vi "Write Results.vi"(8 "error in (no error)":errorcluster, 10 "Results":refnum<class "Acquired Result.lvclass">[](array[class]), 11 "Combined Result in":refnum<class "Combined Result.lvclass">) -> (0 "error out":errorcluster, 3 "Combined Result out":refnum<class "Combined Result.lvclass">)   [LabVIEW 2021, in "Combined Result.lvclass"]
uses:
  Combined Result.lvclass
  Acquired Result/Acquired Result.lvclass
  Combined Result.lvclass/Combined Result.ctl
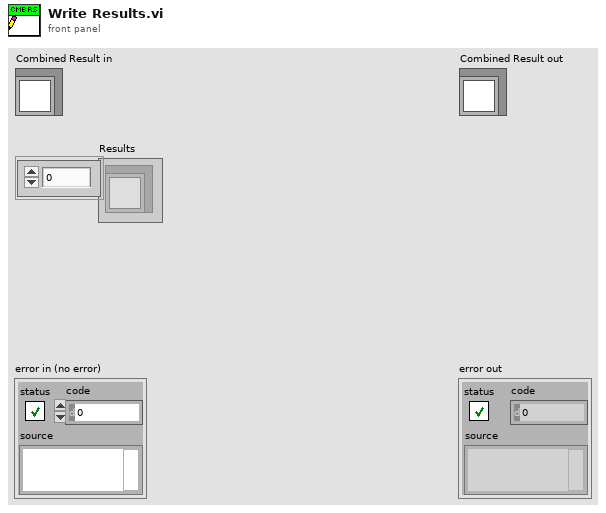
[diagram p1: front panel]
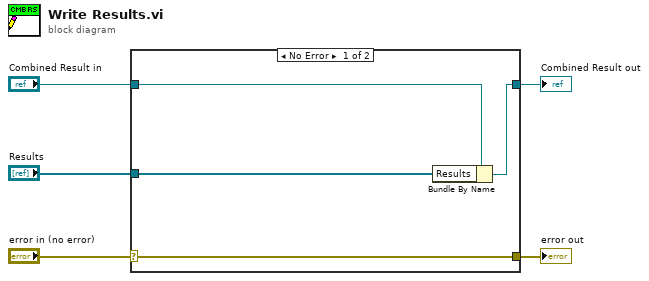
[diagram p0: block diagram]
diagram:
  n1 = case shown="No Error" "error in (no error)" {
    selector: "error in (no error)" -> [w9 w10]
    tunnel: [w9 w10] -> w4
    tunnel: [w7 w11] -> w2
    tunnel: "Combined Result in" -> [w8 w11]
    tunnel: "Results" -> [w6 _]
    frame No Error {
      n2 = Bundle By Name(cluster=w8, "Results"=w6) -> (w7:refnum<class "Combined Result.lvclass">)
    }
    frame Error {
    }
  }
  "error out" <- w4
  "Combined Result out" <- w2
